vi "MatBuilder_Create.vi"(9 "Columns":i32, 11 "Rows":i32) -> (3 "output matrix":T1)   [LabVIEW 2019, in "Trajectory_Library.lvlib"]
doc: "Creates a new matrix with the given dimensions.\n\nInputs:\n - Rows -- Number of rows in the matrix\n - Columns -- Number of columns in the matrix\n\nOutputs:\n - Output Matrix -- The resulting matrix. All values are zero."
uses:
  Trajectory_Library.lvlib
  <vilib>/Analysis/Matrix/Datatypes/RealMatrix.ctl
  <vilib>/Analysis/Matrix/NI_Matrix.lvlib
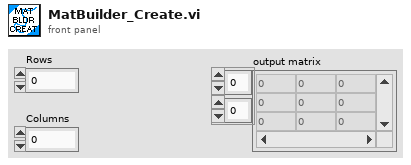
[diagram p1: front panel]
types:
  T1 = typedef "NI_Matrix.lvlib/RealMatrix.ctl" = dbl[][]
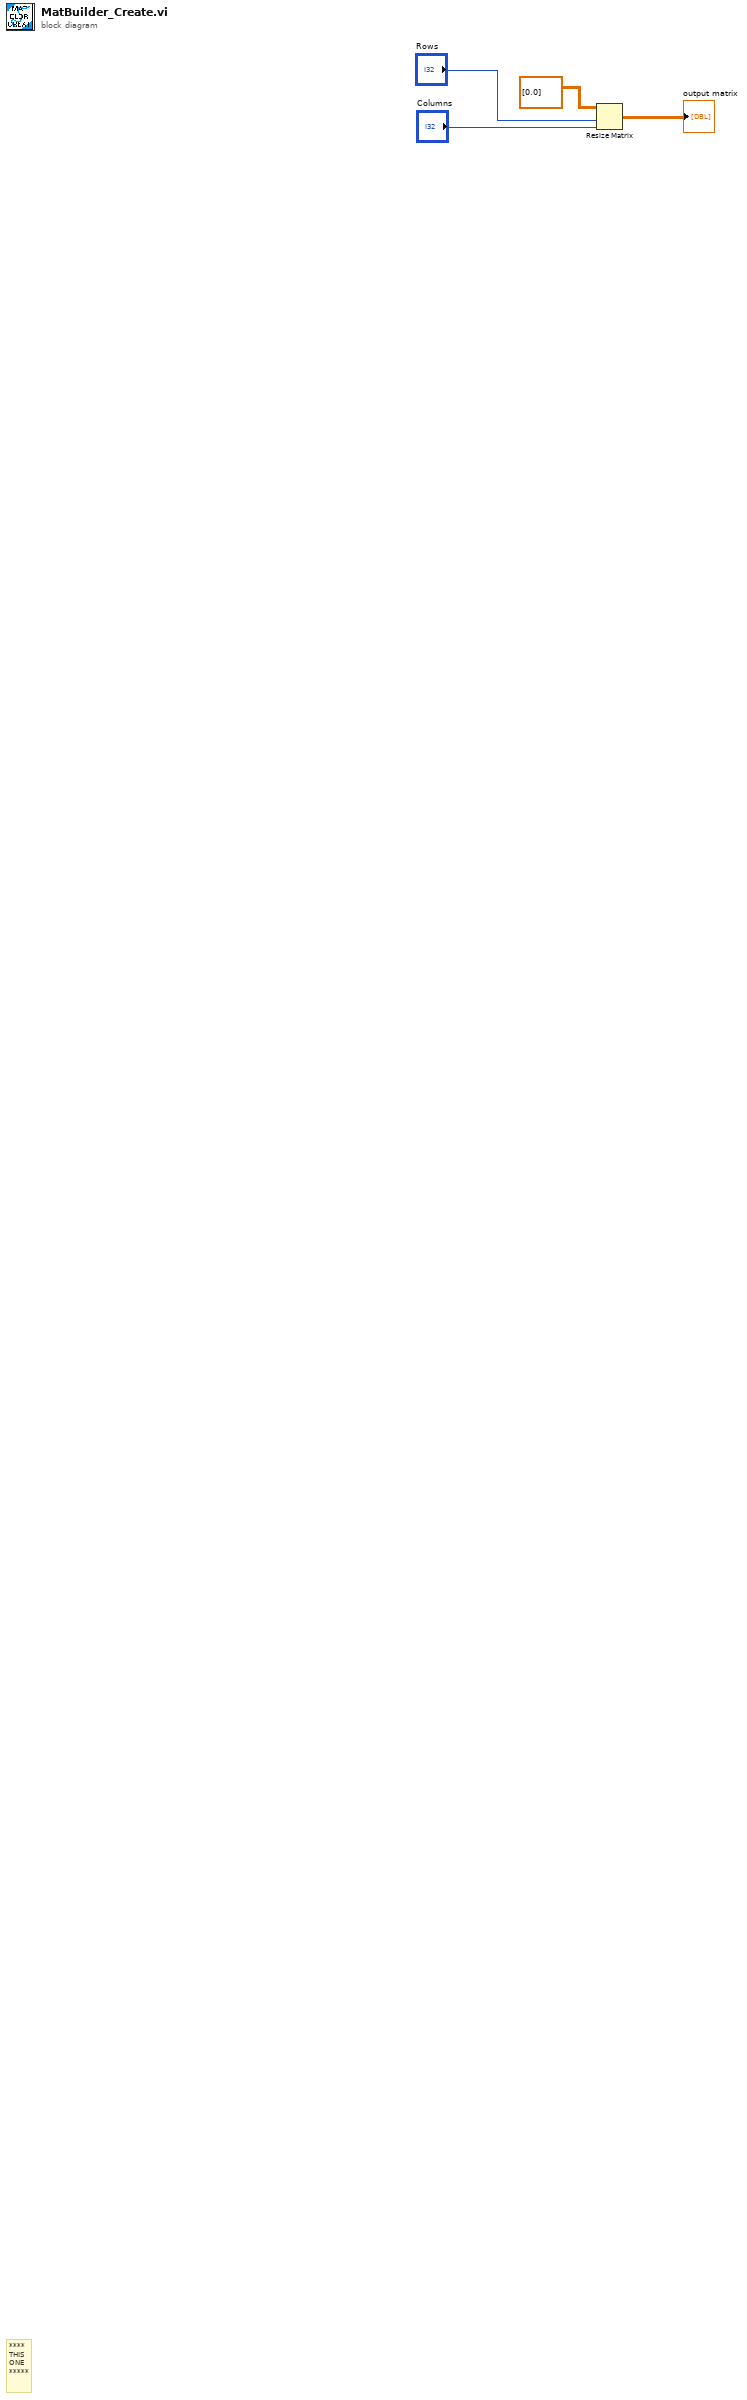
[diagram p0: block diagram]
diagram:
  # "****\nTHIS\nONE\n*****"
  n1 = Resize Matrix(1:"Columns", 2:"Rows", 4:T1 [[0.0]] ("matrix")) -> (0:→"output matrix":T1)
